vi "JSONRPC-BuildMethodInfo.vi"(6 "Example":string, 7 "Description":string="Sends a request to write the value of one or more servers' variables on demand", 8 "Returns":string="JSON", 9 "Params":string, 10 "Method":enum16{"SSE", "GET", "POST"}(ring), 11 "url":string="%s") -> (3 "String":string)   [LabVIEW 2019]
panel:
  # "BuildMethodInfo"
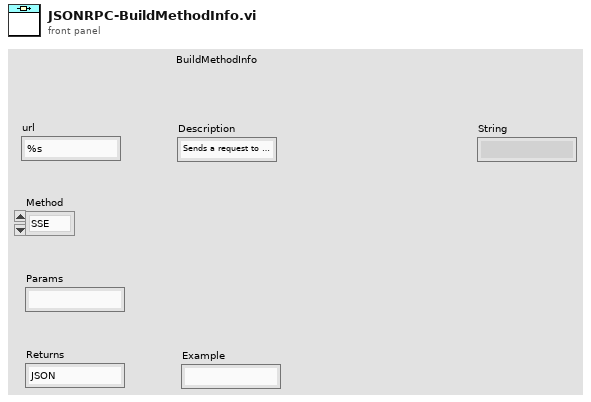
[diagram p1: front panel]
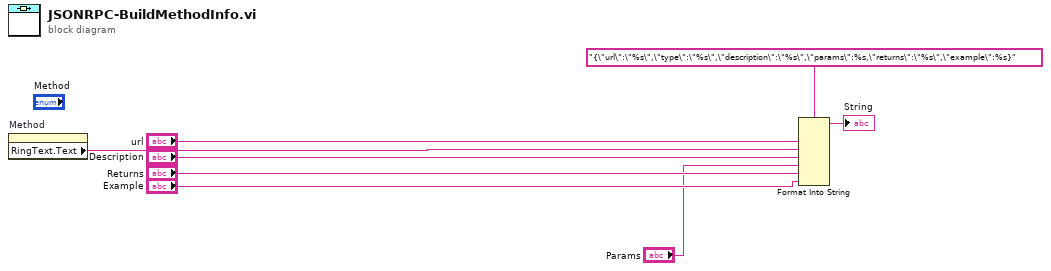
[diagram p0: block diagram]
diagram:
  n1 = property on="Method" class="Enum (strict)"() -> ("RingText.Text"=w2:string)  [unwired: 2 in, 2 out]
  n2 = Format Into String(format string="{\"url\":\"%s\",\"type\":\"%s\",\"description\":\"%s\",\"params\":%s,\"returns\":\"%s\",\"example\":%s}", "url", w2, "Description", "Params", "Returns", "Example") -> (resulting string=→"String":string)  [unwired: 2 in, 1 out]
